vi "Convert_StringData_ToArray.vi"(8 "error in (no error)":errorcluster, 11 "Scikit-learn in":refnum<class "Scikit-learn.lvclass">) -> (0 "error out":errorcluster, 2 "Data":T1, 3 "Scikit-learn out":refnum<class "Scikit-learn.lvclass">)   [LabVIEW 2020, in "Scikit-learn.lvclass"]
doc: "Convert string data to array"
uses:
  Scikit-learn.lvclass
  Scikit-learn.lvclass/Scikit-learn.ctl
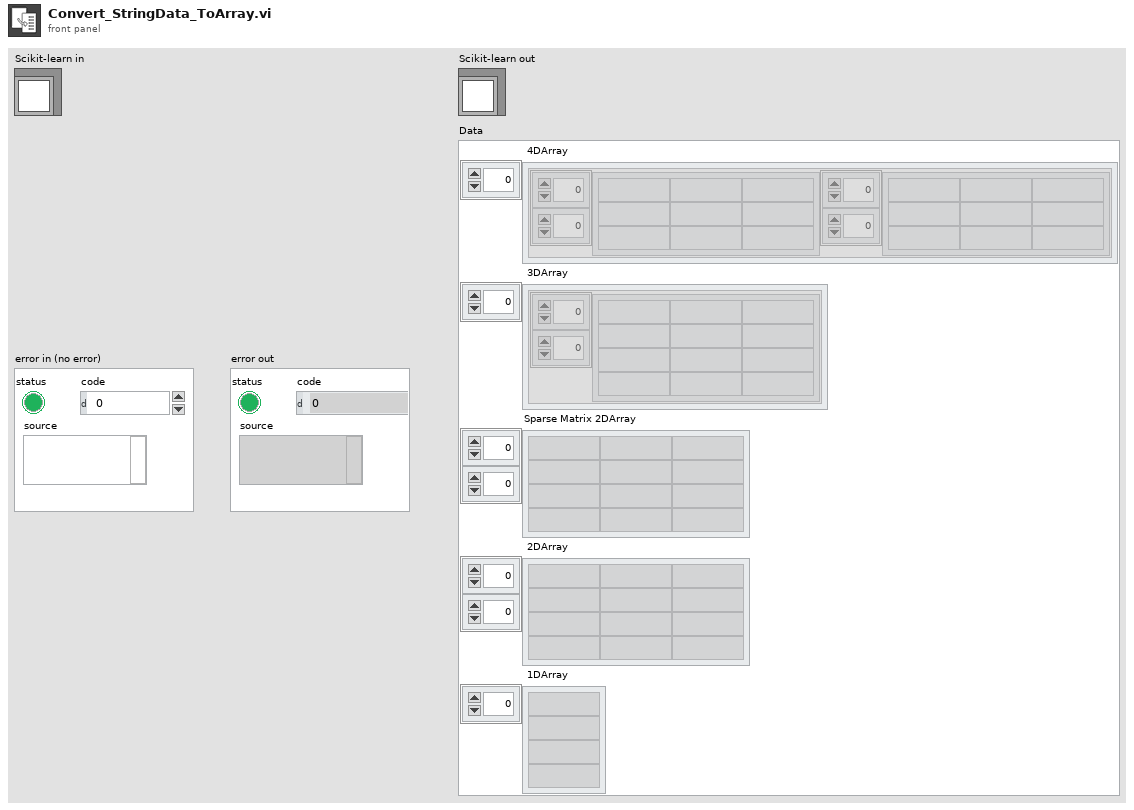
[diagram p1: front panel]
types:
  T1 = cluster{" 4DArray":cluster{"1":string[][], "2":string[][]}[], " 3DArray":cluster{"Tableau":string[][]}[], "Sparse Matrix 2DArray":string[][], " 2DArray":string[][], " 1DArray":string[]}
  T2 = cluster{"String 4DArray":cluster{"1":string[][], "2":string[][]}[], "String 3DArray":cluster{"Tableau":string[][]}[], "String Matrix 2DArray":string[][], "String 2DArray":string[][], "String 1DArray":string[]}
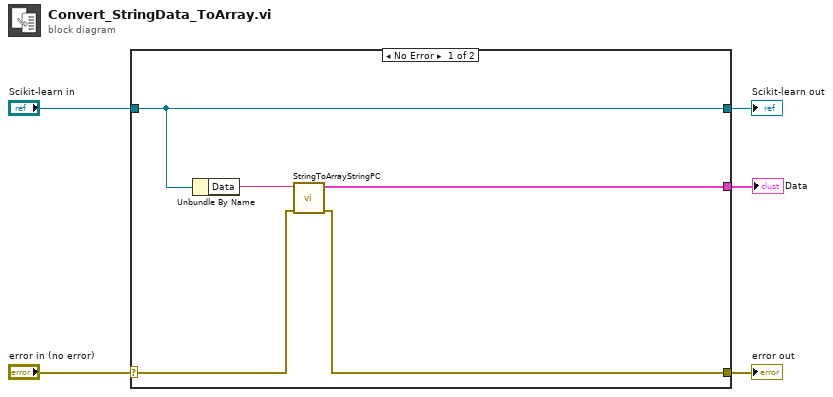
[diagram p0: block diagram]
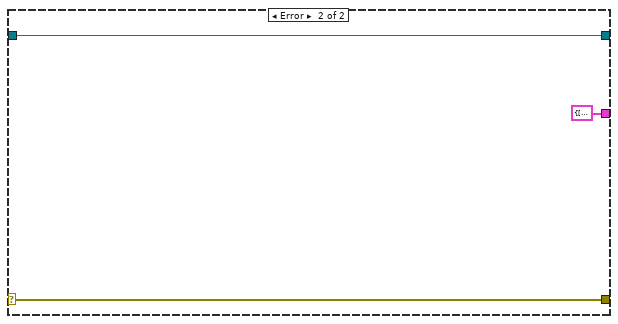
[diagram p2: hidden frame]
diagram:
  n1 = case shown="No Error" "error in (no error)" {
    selector: "error in (no error)" -> [w8 w13]
    tunnel: [w7 w13] -> w4
    tunnel: [w10 w12] -> w2
    tunnel: "Scikit-learn in" -> [w10 w12]
    tunnel: [w6 T2 {"String 4DArray"=[], "String 3DArray"=[], "String Matrix 2DArray"=[], "String 2DArray"=[], "String 1DArray"=[]} ("Data")] -> w1
    frame No Error {
      n2 = Unbundle By Name(w10) -> ("Data"=w9:string)
      n3 = call "StringToArrayStringPC.vi"("sortie d'erreur"=w8, "Return value"=w9) -> ("sortie d'erreur"=w7:errorcluster, "Data"=w6:T1)  [unwired: 8 in]
    }
    frame Error {
    }
  }
  "error out" <- w4
  "Scikit-learn out" <- w2
  "Data" <- w1
